vi "controlo ON OFF.vi"() -> ()   [LabVIEW 2018]
panel:
  out "Boolean":bool
  out "Pipe":bool
  out "Bomba":bool
  in  "stop":bool
  out "Waveform Chart":dynamicdata(graph)
  out "Tank":dbl(slide) scale=0.0..100.0
  out "Nivel depósito":dbl
  in  "Consumo L/s":dbl(slide) scale=0.0..1.0
  in  "Nivel Baixo":dbl
  in  "Nivel alto":dbl
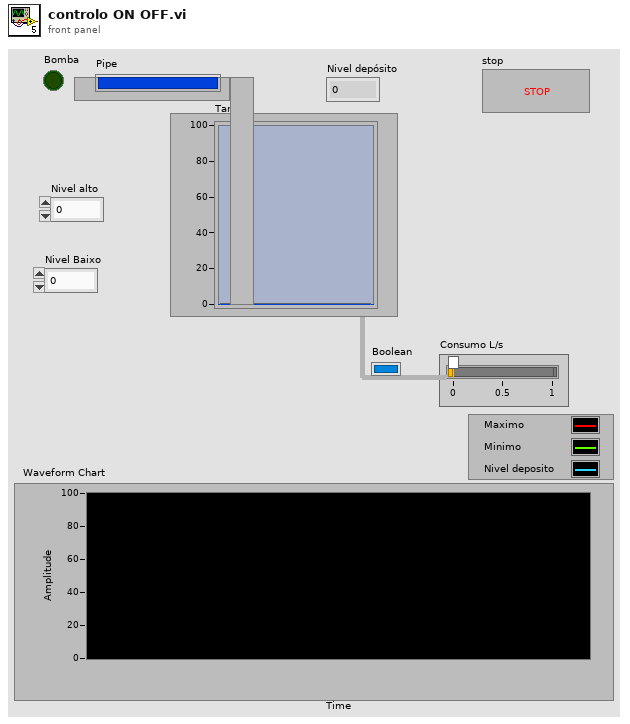
[diagram p1: front panel]
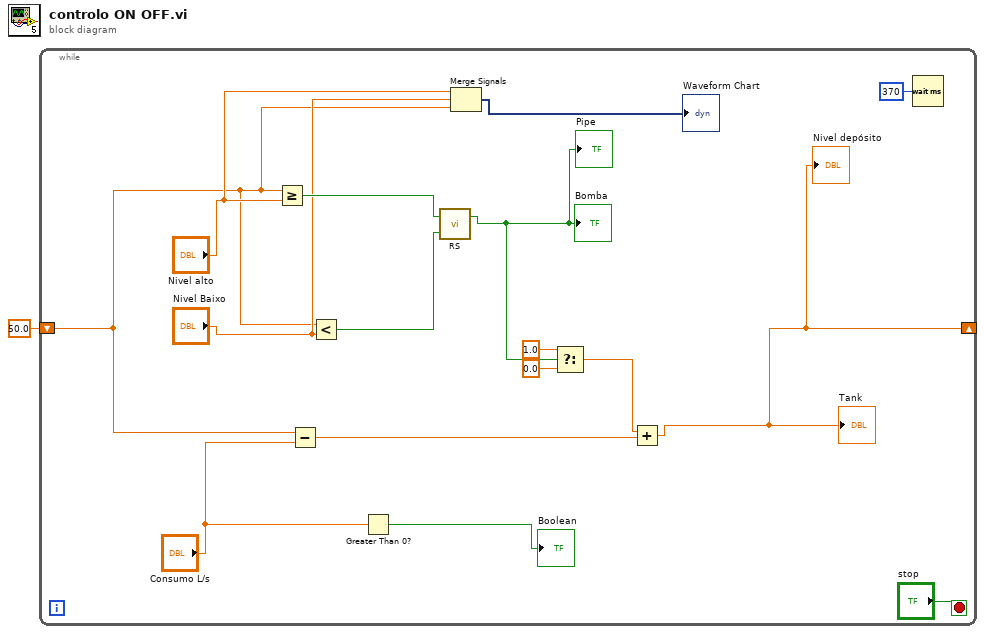
[diagram p0: block diagram]
diagram:
  n1 = while {
    shift-right: [w9] -> _
    shift-left: 50.0 -> [w4]
    stop <- "stop" stop-if-true
    n2 = Greater Or Equal?(x=w4, y="Nivel alto") -> (x >= y?=w15:bool)
    n3 = Subtract(x=w4, y="Consumo L/s") -> (x-y=w10:dbl)
    n4 = Less?(x=w4, y="Nivel Baixo") -> (x < y?=w14:bool)
    n5 = Greater Than 0?(x="Consumo L/s") -> (x > 0?=→"Boolean":bool)
    n6 = call "RS.vi"("SET"=w14, "RESET"=w15) -> ("SAÍDA"=w8:bool)  [unwired: 1 in]
    "Bomba" <- w8
    "Pipe" <- w8
    n7 = Merge Signals("Nivel alto", "Nivel Baixo", w4) -> (→"Waveform Chart":dynamicdata)
    n8 = Select(t=1.0, s=w8, f=0.0) -> (s? t:f=w11:dbl)
    n9 = Add(x=w11, y=w10) -> (x+y=w9:dbl)
    "Tank" <- w9
    "Nivel depósito" <- w9
    n10 = Wait (ms)(milliseconds to wait=u32 370) -> ()  [unwired: 1 out]
  }
